vi "test.vi"   [LabVIEW 2021]
uses:
  <vilib>/Utility/miscctls.llb/LVBoundsTypeDef.ctl
  <vilib>/Utility/miscctls.llb/LVRectTypeDef.ctl
  <vilib>/Utility/miscctls.llb/LVPositionTypeDef.ctl
types:
  T1 = enum32{"Invalid", "Standard", "Closed", "Hidden", "Minimized", "Maximized"}
  T2 = typedef "LVRectTypeDef.ctl" = cluster{"Left":i16, "Top":i16, "Right":i16, "Bottom":i16}
  T3 = typedef "LVBoundsTypeDef.ctl" = cluster{"Width":u32, "Height":u32}
  T4 = typedef "LVPositionTypeDef.ctl" = cluster{"Left":i32, "Top":i32}
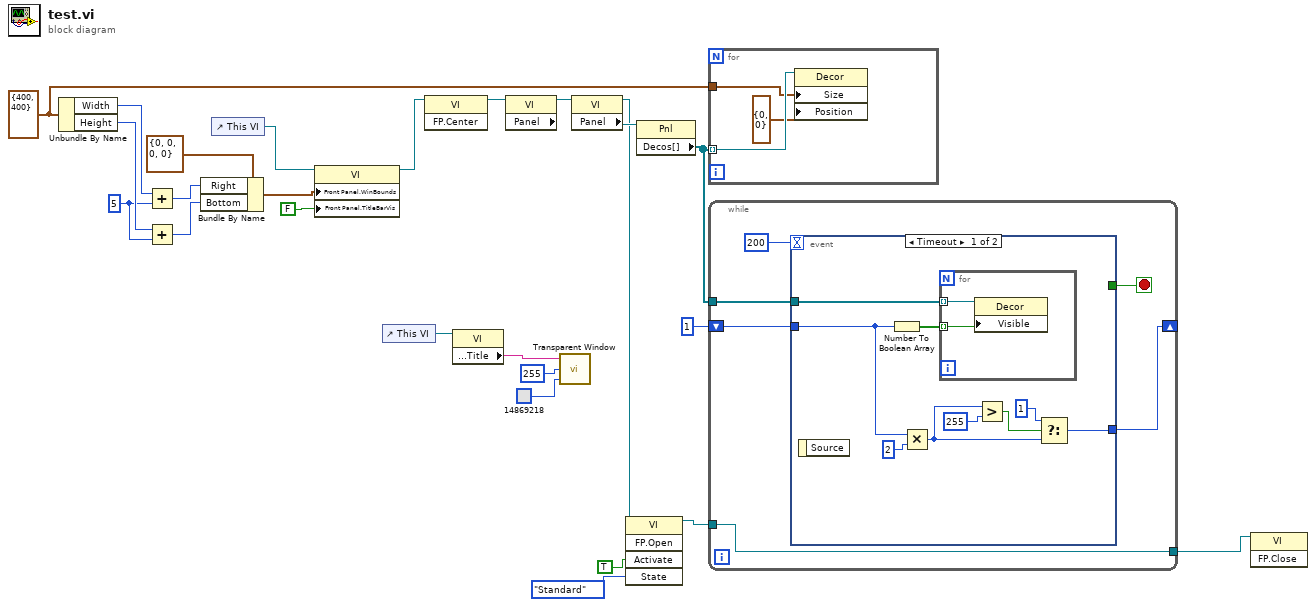
[diagram p0: block diagram]
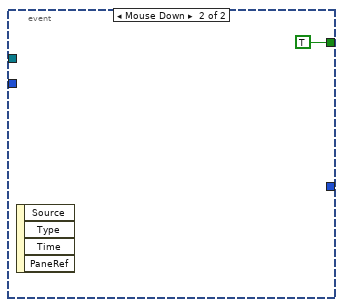
[diagram p2: hidden frame]
diagram:
  w13 = u32 5 ("y")
  w24 = T3 {"Width"=400, "Height"=400} ("Size")
  n1 = Unbundle By Name(w24) -> ("Width"=w17:u32, "Height"=w15:u32)
  n2 = Add(x=w17, y=w13) -> (x+y=w16:u32)
  n3 = Add(x=w15, y=w13) -> (x+y=w14:u32)
  n4 = Bundle By Name(cluster=T2 {"Left"=0, "Top"=0, "Right"=0, "Bottom"=0} ("Front Panel Window:Panel Bounds"), "Right"=w16, "Bottom"=w14) -> (w22:T2)
  n5 = control-ref of="This VI"() -> (w18:refnum<vi>)
  n6 = property class="VI"(reference=w18, "Front Panel.WinBounds"=w22, "Front Panel.TitleBarVis"=FALSE ("Front Panel Window:Title Bar Visible")) -> (reference out=w11:refnum<vi>)  [unwired: 1 in, 1 out]
  n7 = control-ref of="This VI"() -> (w9:refnum<vi>)
  n8 = invoke class="VI" method="FP.Center"(reference=w11) -> (reference out=w10:refnum<vi>)  [unwired: 2 in, 2 out]
  n9 = property class="VI"(reference=w9) -> ("Front Panel.Title"=w6:string)  [unwired: 1 in, 2 out]
  n10 = property class="VI" props=["Panel"](reference=w10) -> (reference out=w19:refnum<vi>)  [unwired: 1 in, 2 out]
  n11 = call "Transparent Window.vi"("crkey"=u32 14869218, "Slide"=u8 255, "window name (\"\")"=w6) -> ()  [unwired: 1 in]
  n12 = property class="VI"(reference=w19) -> (reference out=w5:refnum<vi>, "Panel"=w25:refnum<vi>)  [unwired: 1 in, 1 out]
  n13 = invoke class="VI" method="FP.Open"(reference=w5, "Activate"=TRUE ("Activate?"), "State"=T1."Standard") -> (reference out=w2:refnum<vi>)  [unwired: 2 in, 4 out]
  n14 = property class="Pnl"(reference=w25) -> ("Decos[]"=w21:refnum<vi>[])  [unwired: 1 in, 2 out]
  n15 = for {
    tunnel: w21 -> [w28] mode=indexing
    tunnel: w24 -> [w27]
    n16 = property class="Decor"(reference=w28, "Size"=w27, "Position"=T4 {"Left"=0, "Top"=0}) -> ()  [unwired: 1 in, 2 out]
  }
  n17 = while {
    tunnel: w21 -> [w32]
    shift-right: [w30] -> _
    shift-left: 1 -> [w31]
    tunnel: w2 -> [w29]
    tunnel: [w29] -> w1
    stop <- w33 stop-if-true
    n18 = event shown="[0] Timeout" {
      selector: _ -> [_ _]
      dyn-events: _ -> [_ _]
      timeout: 200 ("Numeric Control") -> [_ _]
      tunnel: [_ TRUE ("Discard?")] -> w33
      tunnel: w32 -> [w43 _]
      tunnel: w31 -> [w35 _]
      tunnel: [w38 _] -> w30
      event Timeout {
        n19 = event-data() -> ()  [unwired: 1 in, 1 out]
        n20 = Number To Boolean Array(number=w35) -> (Boolean array=w36:bool[])
        n21 = Multiply(x=w35, y=2) -> (x*y=w39:i32)
        n22 = for {
          tunnel: w43 -> [w45] mode=indexing
          tunnel: w36 -> [w44] mode=indexing
          n23 = property class="Decor"(reference=w45, "Visible"=w44) -> ()  [unwired: 1 in, 2 out]
        }
        n24 = Greater?(x=w39, y=255) -> (0:w40:bool)
        n25 = Select(t=1, s=w40, f=w39) -> (s? t:f=w38:i32)
      }
      event Mouse Down {
        n26 = event-data() -> ()  [unwired: 1 in, 4 out]
      }
    }
  }
  n27 = invoke class="VI" method="FP.Close"(reference=w1) -> ()  [unwired: 2 in, 3 out]
